vi "Log_Apontamento.vi"() -> ()   [LabVIEW 2018]
uses:
  Global_Telescopio.vi
panel:
  out "Comando":string
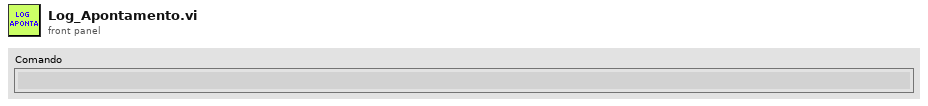
[diagram p1: front panel]
types:
  T1 = enum16{"open", "open or create", "create or replace", "create"}
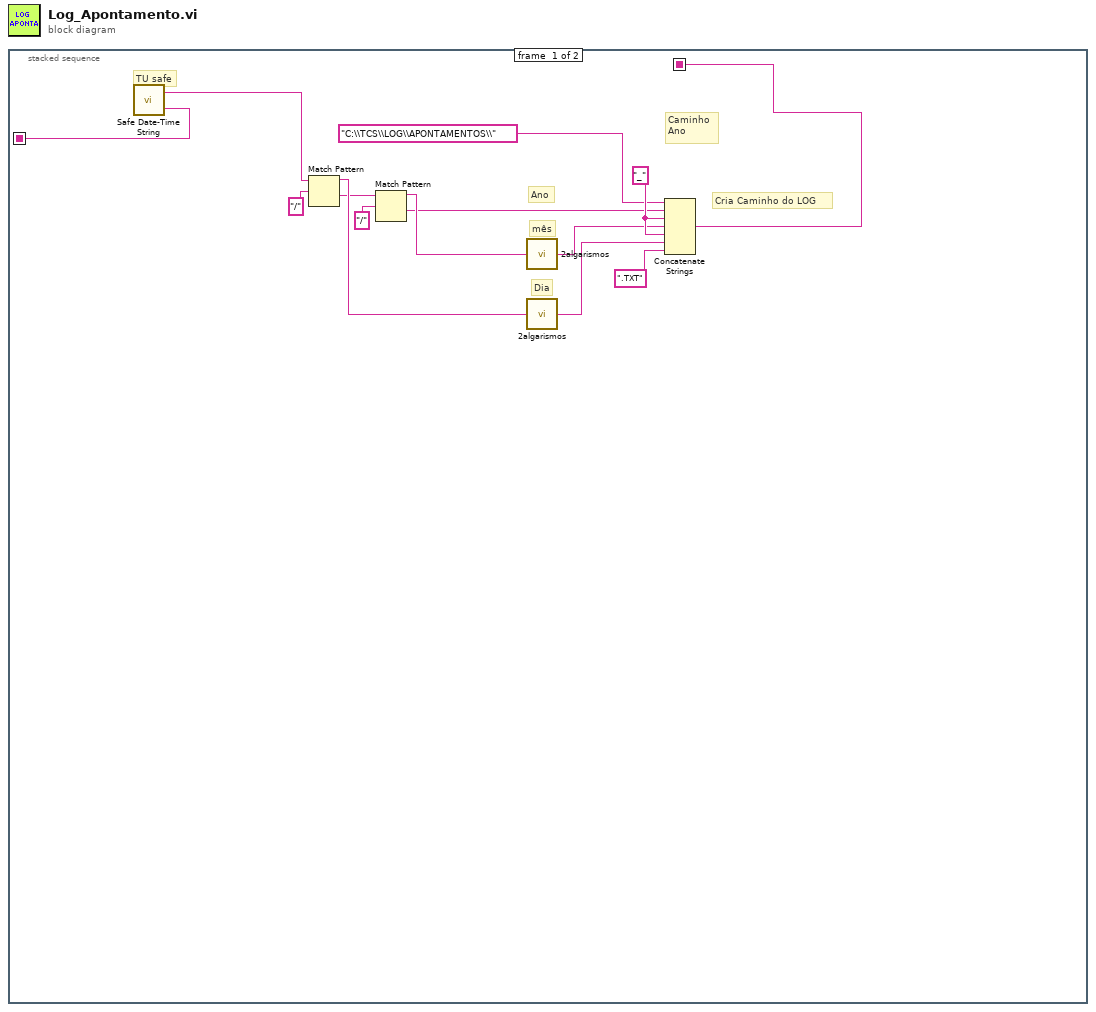
[diagram p0: block diagram]
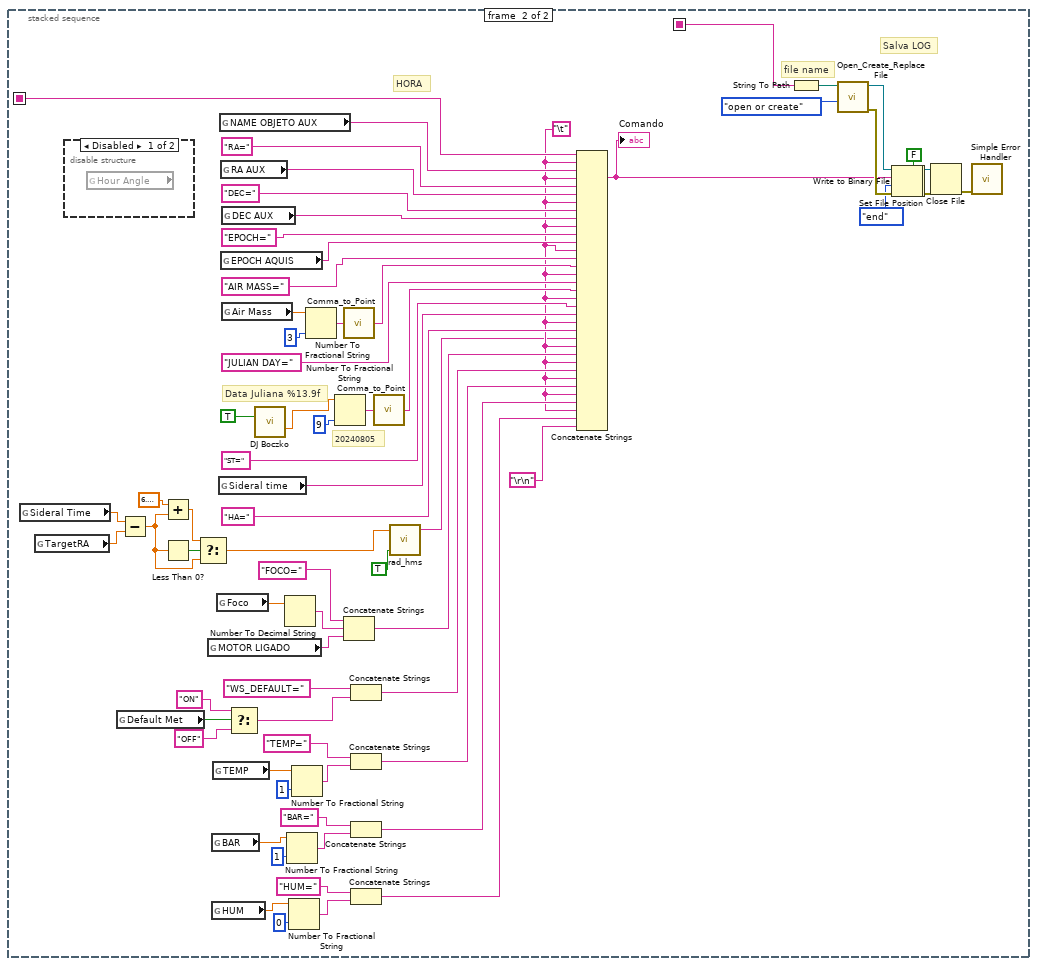
[diagram p2: hidden frame]
diagram:
  n1 = stacked-sequence {
    seq-local: [w3 _] -> [_ w76]
    seq-local: [w2 _] -> [_ w86]
    frame #0 {
      w13 = "_"
      # "TU safe"
      # "Cria Caminho do LOG"
      # "Caminho\nAno"
      # "Ano"
      # "mês"
      # "Dia"
      n2 = call "Safe Date-Time String.vi"() -> ("Safe time string"=w2:string, "Safe date string"=w1:string)  [unwired: 3 in]
      n3 = Match Pattern(string=w1, regular expression="/") -> (before substring=w14:string, after substring=w10:string)  [unwired: 1 in, 2 out]
      n4 = Match Pattern(string=w10, regular expression="/") -> (before substring=w9:string, after substring=w8:string)  [unwired: 1 in, 2 out]
      n5 = call "2algarismos.vi"("entrada"=w9) -> ("saida"=w6:string)
      n6 = call "2algarismos.vi"("entrada"=w14) -> ("saida"=w5:string)
      n7 = Concatenate Strings("C:\\TCS\\LOG\\APONTAMENTOS\\" ("SOMENTE DIRETORIO"), w8, w13, w6, w13, w5, ".TXT" ("regular expression")) -> (w3:string)
    }
    frame #1 {
      w30 = "\t"
      # "20240805"
      # "Data Juliana %13.9f"
      # "HORA"
      # "Salva LOG"
      # "file name"
      n8 = global read "Global_Telescopio.vi" "Sideral Time"() -> (w23:dbl)
      n9 = global read "Global_Telescopio.vi" "TargetRA"() -> (w24:dbl)
      n10 = disable-structure shown="Disabled" {
        frame Disabled {
          n11 = global read "Global_Telescopio.vi" "Hour Angle"() -> ()  [unwired: 1 out]
        }
        frame Enabled {
        }
      }
      n12 = global read "Global_Telescopio.vi" "Default Met"() -> (w18:bool)
      n13 = Subtract(x=w23, y=w24) -> (x-y=w22:dbl)
      n14 = Add(x=6.283185307179586, y=w22) -> (x+y=w26:dbl)
      n15 = Less Than 0?(x=w22) -> (x < 0?=w25:bool)
      n16 = Select(t=w26, s=w25, f=w22) -> (s? t:f=w20:dbl)
      n17 = global read "Global_Telescopio.vi" "MOTOR LIGADO"() -> (w36:string)
      n18 = global read "Global_Telescopio.vi" "BAR"() -> (w41:dbl)
      n19 = global read "Global_Telescopio.vi" "HUM"() -> (w42:dbl)
      n20 = global read "Global_Telescopio.vi" "TEMP"() -> (w37:dbl)
      n21 = global read "Global_Telescopio.vi" "Foco"() -> (w50:dbl)
      n22 = global read "Global_Telescopio.vi" "Sideral time"() -> (w53:string)
      n23 = global read "Global_Telescopio.vi" "NAME OBJETO AUX"() -> (w72:string)
      n24 = global read "Global_Telescopio.vi" "RA AUX"() -> (w70:string)
      n25 = global read "Global_Telescopio.vi" "EPOCH AQUIS"() -> (w66:string)
      n26 = global read "Global_Telescopio.vi" "DEC AUX"() -> (w68:string)
      n27 = global read "Global_Telescopio.vi" "Air Mass"() -> (w63:dbl)
      n28 = Select(t="ON", s=w18, f="OFF") -> (s? t:f=w15:string)
      n29 = call "DJ Boczko.vi"("TRUE = Hora Local\nFALSE = UT"=TRUE ("TRUE = Hora Local\nFALSE = UT")) -> ("Dia Juliano"=w59:dbl)  [unwired: 6 in, 8 out]
      n30 = Number To Decimal String(number=w50) -> (decimal integer string=w51:string)  [unwired: 1 in]
      n31 = Number To Fractional String(number=w41, precision (6)=i16 1) -> (F-format string=w48:string)  [unwired: 2 in]
      n32 = Number To Fractional String(number=w42, precision (6)=i16 0) -> (F-format string=w49:string)  [unwired: 2 in]
      n33 = Number To Fractional String(number=w37, precision (6)=i16 1) -> (F-format string=w46:string)  [unwired: 2 in]
      n34 = Number To Fractional String(number=w63, precision (6)=i16 3) -> (F-format string=w65:string)  [unwired: 2 in]
      n35 = Number To Fractional String(number=w59, precision (6)=i16 9) -> (F-format string=w60:string)  [unwired: 2 in]
      n36 = call "Comma_to_Point.vi"("Lat_A"=w65) -> ("Saída"=w61:string)
      n37 = Concatenate Strings("FOCO=", w51, w36) -> (w34:string)
      n38 = Concatenate Strings("WS_DEFAULT=" ("string"), w15) -> (w33:string)
      n39 = Concatenate Strings("TEMP=" ("string"), w46) -> (w32:string)
      n40 = Concatenate Strings("BAR=" ("string"), w48) -> (w31:string)
      n41 = Concatenate Strings("HUM=" ("string"), w49) -> (w29:string)
      n42 = call "Comma_to_Point.vi"("Lat_A"=w60) -> ("Saída"=w55:string)
      n43 = call "rad_hms.vi"("TRUE=HORA\nFALSE=GRAU"=TRUE ("TRUE=HORA\nFALSE=GRAU"), "Radiano"=w20) -> ("Hora/Graus Texto Decimal"=w19:string)  [unwired: 3 in]
      n44 = Concatenate Strings(w86, w30, w72, w30, "RA=", w70, w30, "DEC=", w68, w30, "EPOCH=", w66, w30, "AIR MASS=", w61, w30, "JULIAN DAY=", w55, w30, "ST=", w53, w30, "HA=", w19, w30, w34, w30, w33, w30, w32, w30, w31, w30, w29, "\r\n") -> (w77:string)
      "Comando" <- w77
      n45 = String To Path(string=w76) -> (path=w78:path)
      n46 = call <vilib>:"Open_Create_Replace File.vi"("function (open:0)"=T1."open or create", "file path"=w78) -> ("error out"=w81:errorcluster, "refnum"=w84:refnum<file>)  [unwired: 6 in, 2 out]
      n47 = Set File Position(refnum=w84, from (0:start)=enum16{"start", "end", "current"}."end" ("pos mode (0:2)"), error in=w81) -> (refnum out=w75:refnum<file>, error out=w74:errorcluster)  [unwired: 1 in]
      n48 = Write to Binary File(file (use dialog)=w75, data=w77, error in=w74, 5:FALSE ("prepend array or string size? (T)")) -> (refnum out=w83:refnum<file>, error out=w82:errorcluster)  [unwired: 2 in, 1 out]
      n49 = Close File(refnum=w83, error in=w82) -> (error out=w85:errorcluster)  [unwired: 1 out]
      n50 = call <vilib>:"Simple Error Handler.vi"("error in (no error)"=w85) -> ()  [unwired: 4 in, 5 out]
    }
  }
